vi "Proyecto Puntos extra Pualasin Carlos.vi"() -> ()   [LabVIEW 2025]
uses:
  <vilib>/MakerHub/LINX/Public/Peripherals/Digital/Digital Read 1 Chan.vi
  <vilib>/MakerHub/LINX/Public/Peripherals/Analog/Analog Read 1 Chan.vi
  <vilib>/MakerHub/LINX/Public/Peripherals/Digital/Digital Read N Chans.vi
  <vilib>/MakerHub/LINX/Public/Peripherals/Analog/Analog Read N Chans.vi
  <vilib>/MakerHub/LINX/Private/Local IO/LinxDigitalRead.vi
  <vilib>/MakerHub/LINX/Public/Utilities/Check Channel.vi
  <vilib>/MakerHub/LINX/Private/Local IO/LinxAnalogRead.vi
  <vilib>/MakerHub/LINX/Public/Utilities/Open Serial.vi
  <vilib>/MakerHub/LINX/Private/Utilties/Generate Error.vi
  <vilib>/MakerHub/LINX/LMH-LINX.lvlib
panel:
  in  "Serial Port":refnum<visa-resource-name>="N/A"
  in  "stop":bool
  out "INCENDIO":bool
  out "TEMPERATURA ALTA":bool
  out "POSIBLE FUEGO":bool
  out "NORMAL":bool
  out "Temperatura (°C)":dbl
  out "Temperatura Ambiente.":dbl(slide) scale=20.0..25.0
  # "SISTEMA CONTRA PREVENCION DE INCENDIOS"
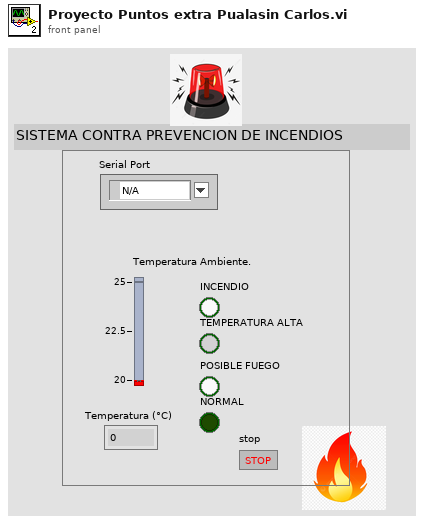
[diagram p1: front panel]
types:
  T1 = typedef "LMH-LINX.lvlib/LINX Ref.ctl" = cluster{"IO":T2, "Interface":T3, "LINX Device Config":T4}
  T2 = typedef "LMH-LINX.lvlib/Platform.ctl" = enum16{"Remote", "Local"}
  T3 = typedef "LMH-LINX.lvlib/Interface.ctl" = enum16{"Serial", "TCP"}
  T4 = typedef "LMH-LINX.lvlib/Device.lvlib/LINX Device Config.ctl" = cluster{"Interface":T3, "COM Port":refnum<visa-resource-name>, "TCP Configuration":T5, "Device Family":u8, "Device ID":u8, "Device Name":string, "TCP Ref":refnum<k5>, "Channels":T6}
  T5 = typedef "LMH-LINX.lvlib/Device.lvlib/TCP Config.ctl" = cluster{"IP Address":string, "Port":u16}
  T6 = typedef "LMH-LINX.lvlib/Channels.ctl" = cluster{"DI":u8[], "DO":u8[], "AI":u8[], "AO":u8[], "PWM":u8[], "QE":u8[], "UART":u8[], "I2C 2":u8[], "SPI":u8[], "CAN":u8[], "Servo":u8[], "AI Ref (V)":dbl, "AI Resolution (Bits)":u8, "AO Ref (V)":dbl, "AO Resolution (Bits)":u8}
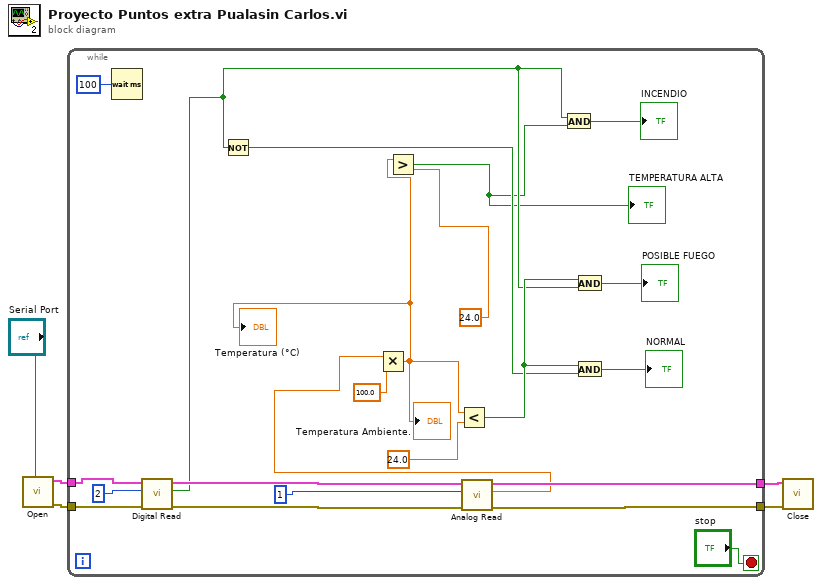
[diagram p0: block diagram]
diagram:
  n1 = call-poly <vilib>:"Open.vi"("Serial Port"="Serial Port") -> ("Error Out"=w4:errorcluster, "LINX Resource"=w5:T1)  [unwired: 8 in, 1 out]
  n2 = while {
    tunnel: w5 -> [w21]
    tunnel: w4 -> [w20]
    tunnel: [w16] -> w3
    tunnel: [w14] -> w2
    stop <- "stop" stop-if-true
    n3 = Wait (ms)(milliseconds to wait=u32 100) -> ()  [unwired: 1 out]
    n4 = call-poly <vilib>:"Digital Read.vi"("Error In"=w20, "DI Channel"=u8 2, "LINX Resource"=w21) -> ("Error Out"=w15:errorcluster, "DI Value"=w11:bool, "LINX Resource"=w17:T1)  [unwired: 6 in]
    n5 = Not(x=w11) -> (.not. x?=w9:bool)
    n6 = call-poly <vilib>:"Analog Read.vi"("Error In"=w15, "Analog Channel"=u8 1, "LINX Resource"=w17) -> ("Error Out"=w14:errorcluster, "Voltage"=w7:dbl, "LINX Resource"=w16:T1)  [unwired: 5 in, 1 out]
    n7 = Multiply(x=w7, y=100.0) -> (x*y=w8:dbl)
    "Temperatura Ambiente." <- w8
    "Temperatura (°C)" <- w8
    n8 = Greater?(x=w8, y=24.0) -> (0:w6:bool)
    "TEMPERATURA ALTA" <- w6
    n9 = Less?(x=w8, y=24.0) -> (x < y?=w24:bool)
    n10 = And(x=w11, y=w6) -> (x .and. y?=→"INCENDIO":bool)
    n11 = And(x=w24, y=w11) -> (x .and. y?=→"POSIBLE FUEGO":bool)
    n12 = And(x=w24, y=w9) -> (x .and. y?=→"NORMAL":bool)
  }
  n13 = call <vilib>:"Close.vi"("Error In"=w2, "LINX Resource"=w3) -> ()  [unwired: 9 in, 1 out]
